vi "GLOBALS.vi"() -> ()   [LabVIEW 2019]
uses:
  Utility/Globals_IO.ctl
panel:
  in  "I/O":T1
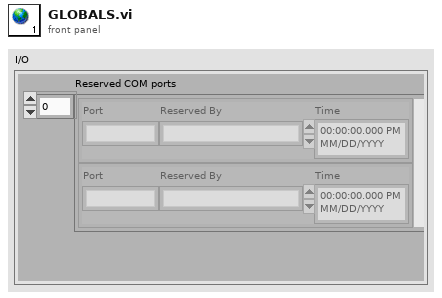
[diagram p1: front panel]
types:
  T1 = typedef "Globals_IO.ctl" = cluster{"Reserved COM ports":cluster{"Port":string, "Reserved By":string, "Time":timestamp}[]}
diagram:
